vi "Flush Target Messages.vi"(8 "error in (no error)":errorcluster, 10 "Mail Strategy In":refnum<class "Mail Strategy.lvclass">, 11 "Map Tree Queue Messenger in":refnum<class "Map Tree Queue Messenger.lvclass">) -> (0 "error out":errorcluster, 2 "Flushed Messages":refnum<class "Message.lvclass">[](array[class]), 3 "Map Tree Queue Messenger out":refnum<class "Map Tree Queue Messenger.lvclass">)   [LabVIEW 2019, in "Map Tree Queue Messenger.lvclass"]
uses:
  Map Tree Queue Messenger.lvclass
  C:/Users/User/Desktop/Bussiness/Multi SPIM/General Library/Ancestor Class/Messenger/Messenger Map Composite/Messenger Map Composite.lvclass
  Ancestor Class/Messenger/Mail Strategy/Mail Strategy.lvclass
  Ancestor Class/Message/Message.lvclass
  Simple Tree Queue Mailman/Simple Tree Queue Mailman.lvclass
  C:/Users/User/Desktop/Bussiness/Multi SPIM/General Library/Ancestor Class/Messenger/Mail Strategy/Mail Strategy.lvclass
  Ancestor Class/Messenger/Messenger Map Composite/Messenger Map Composite.lvclass/Messenger Map Composite.ctl
  Simple Tree Queue Mailman/Simple Tree Queue Mailman.lvclass/Simple Tree Queue Mailman.ctl
  Map Tree Queue Messenger.lvclass/Map Tree Queue Messenger.ctl
  Simple Tree Queue Mailman/Public Data/Write Address Recursive Access.vi
  Ancestor Class/Messenger/Messenger Map Composite/Public Data/Read Child Nodes.vi
  Ancestor Class/Messenger/Messenger/Messenger.lvclass
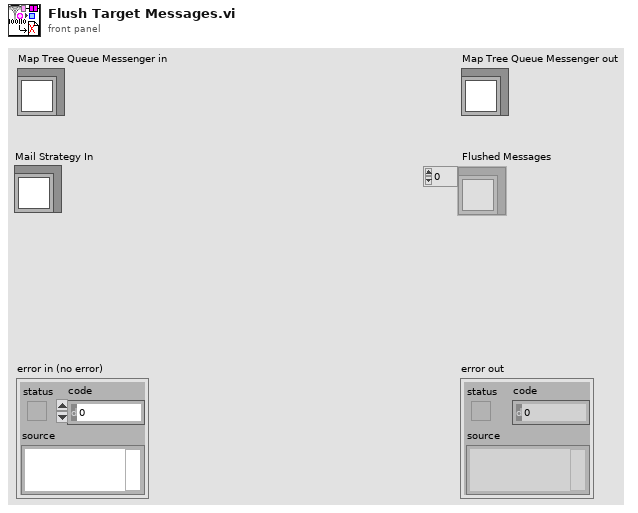
[diagram p1: front panel]
types:
  T1 = typedef "Message Queue.ctl" = refnum<queue>
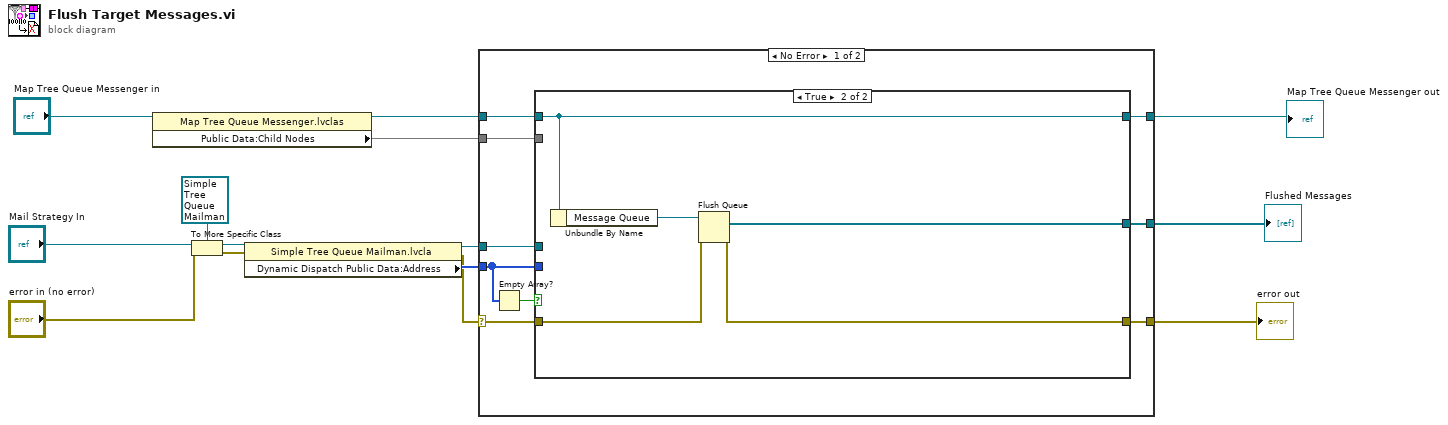
[diagram p0: block diagram]
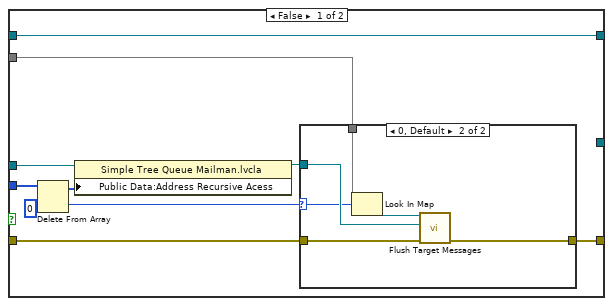
[diagram p2: hidden frame]
diagram:
  n1 = property class="Map Tree Queue Messenger.lvclas"(reference="Map Tree Queue Messenger in") -> (reference out=w10:refnum<class "Map Tree Queue Messenger.lvclass">, "Public Data:Child Nodes"=w9:map{i64, refnum<class "Messenger.lvclass">})  [unwired: 1 in, 1 out]
  n2 = To More Specific Class(target class=refnum<class "Simple Tree Queue Mailman.lvclass"> refnum ("Array Location Mailman.lvclass"), reference="Mail Strategy In", error in="error in (no error)") -> (specific class reference=w13:refnum<class "Simple Tree Queue Mailman.lvclass">, error out=w14:errorcluster)
  n3 = property class="Simple Tree Queue Mailman.lvcla"(reference=w13, error in=w14) -> (reference out=w8:refnum<class "Simple Tree Queue Mailman.lvclass">, error out=w11:errorcluster, "Dynamic Dispatch Public Data:Address"=w12:i32[])
  n4 = case shown="No Error" w11 {
    selector: w11 -> [w19 w46]
    tunnel: w10 -> [w22 w47]
    tunnel: [w21 w47] -> w2
    tunnel: [w18 w46] -> w3
    tunnel: w12 -> [w20 _]
    tunnel: w9 -> [w17 _]
    tunnel: w8 -> [w16 _]
    tunnel: [w15 _] -> w1
    frame No Error {
      n5 = Empty Array?(array=w20) -> (empty?=w23:bool)
      n6 = case shown="True" w23 {
        tunnel: w22 -> [w33 w45]
        tunnel: [w33 w45] -> w21
        tunnel: w20 -> [w32 _]
        tunnel: w19 -> [w30 w43]
        tunnel: [w29 w42] -> w18
        tunnel: w17 -> [w28 _]
        tunnel: w16 -> [w27 _]
        tunnel: [_ w41] -> w15
        frame False {
          n7 = Delete From Array(array=w32, index=0) -> (deleted portion=w24:i32, array with subset deleted=w26:i32[])  [unwired: 1 in]
          n8 = property class="Simple Tree Queue Mailman.lvcla"(reference=w27, "Public Data:Address Recursive Acess"=w26) -> (reference out=w25:refnum<class "Simple Tree Queue Mailman.lvclass">)  [unwired: 1 in, 1 out]
          n9 = case shown="0, Default" w24 {
            selector: w24 -> [_ w35]
            tunnel: w30 -> [w34 w37]
            tunnel: [w34 w36] -> w29
            tunnel: w28 -> [_ w40]
            tunnel: w25 -> [_ w38]
            frame -2147483648..-1 {
            }
            frame 0, Default {
              n10 = Look In Map(map=w40, key=w35) -> (value=w39:refnum<class "Messenger.lvclass">)  [unwired: 1 in, 1 out]
              n11 = call-dynamic "Flush Target Messages.vi"("error in (no error)"=w37, "Mail Strategy In"=w38, "Messenger in"=w39) -> ("error out"=w36:errorcluster)  [unwired: 6 in, 2 out]
            }
          }
        }
        frame True {
          n12 = Unbundle By Name(w45) -> ("Message Queue"=w44:T1)
          n13 = Flush Queue(queue=w44, error in (no error)=w43) -> (remaining elements=w41:refnum<class "Message.lvclass">[], error out=w42:errorcluster)  [unwired: 1 out]
        }
      }
    }
    frame Error {
    }
  }
  "error out" <- w3
  "Map Tree Queue Messenger out" <- w2
  "Flushed Messages" <- w1
